vi "Beatback_PID.vi"(0 "Enable":bool, 1 "Setpoint":sgl, 2 "ProcessVariable":sgl, 5 "Kp":sgl, 6 "Ki":sgl, 7 "Kd":sgl, 8 "OutLLim":sgl=-inf, 10 "OutULim":sgl=inf, 11 "BeatbackDiff":sgl, 12 "IntLLim":sgl=-inf, 13 "Reinitialize? (F)":bool, 14 "IntULim":sgl=inf, 15 "dt [s]":sgl=-1.0, 16 "DerLLim":sgl=-inf, 18 "DerULim":sgl=inf) -> (20 "Output":sgl, 21 "PEffort":sgl, 22 "IEffort":sgl, 23 "DEffort":sgl, 24 "Error":sgl, 25 "dt out [s]":sgl)   [LabVIEW 2015, in "ECS-RT.lvlib"]
doc: "This PID controller has 'beatback' functionality, which is particularly useful in a multiple-controller system where a single controller is chosen as the desired output. Beatback allows the difference between the controller's output and chosen output to be accounted for in the controller's integral component, allowing a 'bumpless' transition. This difference, or 'BeatbackDiff,' is calculated externally and connected via a feedback node."
uses:
  ECS-RT.lvlib
  <vilib>/Analysis/3filter.llb/Filter Passband Type.ctl
  <vilib>/ptbypt/NI_PtbyPt.lvlib
  <vilib>/Analysis/NI_AALBase.lvlib
panel:
  in  "Filter Cutoff [Hz]":sgl=25.0 format="%0.3f"
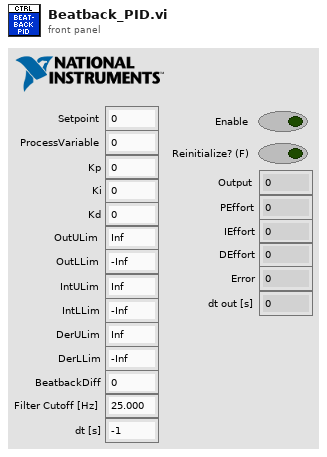
[diagram p1: front panel]
types:
  T1 = typedef "NI_AALBase.lvlib/Filter Passband Type.ctl" = enum32{"Lowpass", "Highpass", "Bandpass", "Bandstop"}
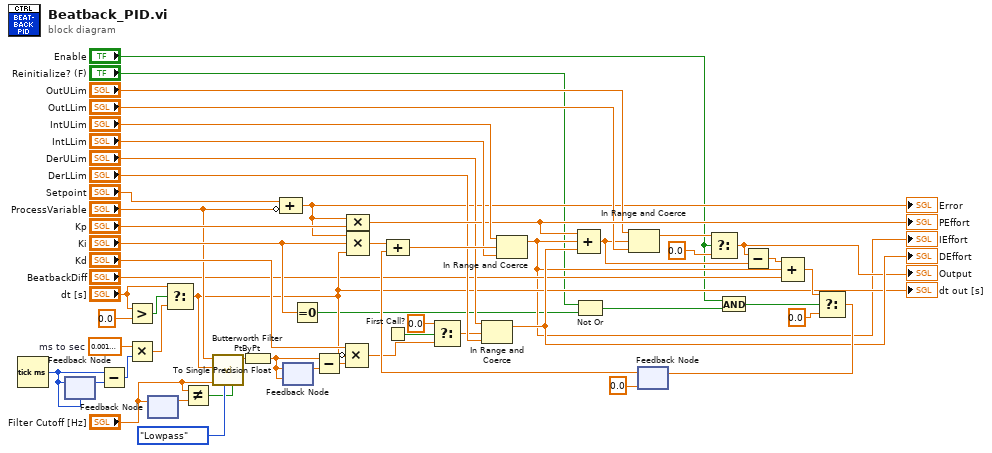
[diagram p0: block diagram]
diagram:
  w22 = sgl 0.001  # ms to sec
  n1 = Tick Count (ms)() -> (millisecond timer value=w24:u32)
  n2 = feedback #1(w24) -> (w25:u32)
  n3 = feedback-in #1(w24) -> ()
  n4 = Subtract(x=w24, y=w25) -> (x-y=w21:u32)
  n5 = Greater?(x="dt [s]", y=sgl 0.0) -> (0:w27:bool)
  n6 = Multiply(x=w22, y=w21) -> (x*y=w23:sgl)
  n7 = feedback #2() -> (w11:sgl)  [unwired: 1 in]
  n8 = feedback-in #2("Filter Cutoff [Hz]") -> ()
  n9 = Select(t="dt [s]", s=w27, f=w23) -> (s? t:f=w12:sgl)
  "dt out [s]" <- w12
  n10 = Not Equal?(x="Filter Cutoff [Hz]", y=w11) -> (x != y?=w9:bool)
  n11 = call <vilib>:"Butterworth Filter PtByPt.vi"("initialize"=w9, "filter type"=Filter_Passband_Type."Lowpass", "low cutoff freq: fl"="Filter Cutoff [Hz]", "sampling freq: fs"=w12, "x"="ProcessVariable") -> ("Filtered x"=w15:dbl)  [unwired: 4 in, 1 out]
  n12 = To Single Precision Float(number=w15) -> (single precision float=w8:sgl)
  n13 = Compound Arithmetic op=ADD("Setpoint", invert "ProcessVariable") -> (w17:sgl)
  "Error" <- w17
  n14 = feedback #3(w8) -> (w29:sgl)
  n15 = feedback-in #3(w8) -> ()
  n16 = Equal To 0?(x="Ki") -> (x = 0?=w5:bool)
  n17 = Subtract(x=w8, y=w29) -> (x-y=w30:sgl)
  n18 = Compound Arithmetic op=MULTIPLY("Kd", invert w12, w30) -> (w18:sgl)
  n19 = Compound Arithmetic op=MULTIPLY(w17, "Kp") -> (w44:sgl)
  "PEffort" <- w44
  n20 = Compound Arithmetic op=MULTIPLY(w17, "Ki", w12) -> (w53:sgl)
  n21 = First Call?() -> (First Call?: T/F=w16:bool)
  n22 = Select(t=sgl 0.0, s=w16, f=w18) -> (s? t:f=w19:sgl)
  n23 = In Range and Coerce(upper limit="DerULim", x=w19, lower limit="DerLLim") -> (coerced(x)=w34:sgl)  [unwired: 1 out]
  "DEffort" <- w34
  n24 = Not Or(1:w5, 2:"Reinitialize? (F)") -> (0:w3:bool)
  n25 = feedback #4(sgl 0.0) -> (w51:sgl)
  n26 = Compound Arithmetic op=ADD(w53, w51) -> (w47:sgl)
  n27 = In Range and Coerce(upper limit="IntULim", x=w47, lower limit="IntLLim") -> (coerced(x)=w6:sgl)  [unwired: 1 out]
  "IEffort" <- w6
  n28 = Compound Arithmetic op=ADD(w44, w6, w34) -> (w38:sgl)
  n29 = In Range and Coerce(upper limit="OutULim", x=w38, lower limit="OutLLim") -> (coerced(x)=w39:sgl)  [unwired: 1 out]
  n30 = Select(t=w39, s="Enable", f=sgl 0.0) -> (s? t:f=w33:sgl)
  "Output" <- w33
  n31 = And(x="Enable", y=w3) -> (x .and. y?=w1:bool)
  n32 = Subtract(x=w33, y=w38) -> (x-y=w37:sgl)
  n33 = Compound Arithmetic op=ADD(w37, w6, "BeatbackDiff") -> (w41:sgl)
  n34 = Select(t=w41, s=w1, f=sgl 0.0) -> (s? t:f=w48:sgl)
  n35 = feedback-in #4(w48) -> ()
